vi "Get Target Method Path.vi"(7 "App Inst":refnum<vi>, 8 "error in (no error)":errorcluster, 10 "Target Method":string, 11 "Target Actor Path":path) -> (0 "error out":errorcluster, 2 "Target Method Path":path)   [LabVIEW 2020, in "Message Rescripter.lvlib"]
uses:
  Message Rescripter.lvlib
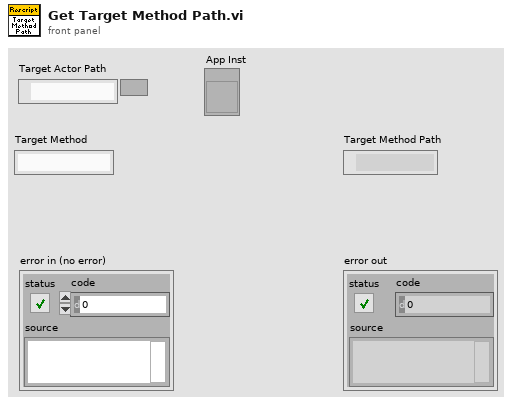
[diagram p1: front panel]
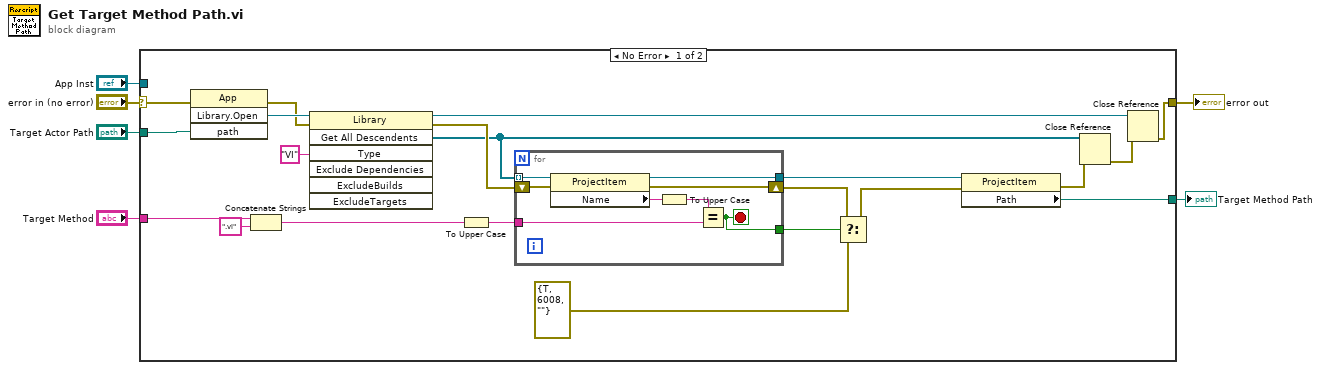
[diagram p0: block diagram]
diagram:
  n1 = case shown="No Error" "error in (no error)" {
    selector: "error in (no error)" -> [w14 w36]
    tunnel: "Target Actor Path" -> [w27 _]
    tunnel: "Target Method" -> [w24 _]
    tunnel: [w18 _] -> w4
    tunnel: [w15 w36] -> w2
    tunnel: "App Inst" -> [_ _]
    frame No Error {
      n2 = invoke class="App" method="Library.Open"(error in=w14, "path"=w27) -> (error out=w13:errorcluster, "Open Library"=w26:refnum<vi>)  [unwired: 2 in, 2 out]
      n3 = Concatenate Strings(w24, ".vi" ("string")) -> (w8:string)
      n4 = invoke class="Library" method="Get All Descendents"(reference=w26, error in=w13, "Type"="VI") -> (reference out=w17:refnum<vi>, error out=w21:errorcluster, "All Descendents"=w19:refnum<vi>[])  [unwired: 4 in, 4 out]
      n5 = To Upper Case(1:w8) -> (0:w23:string)
      n6 = for {
        tunnel: w19 -> [w34] mode=indexing
        tunnel: [w33] -> w22
        tunnel: w23 -> [w32]
        shift-right: [w30] -> w11
        shift-left: w21 -> [w31]
        tunnel: [w29] -> w12
        stop <- w29 stop-if-true
        n7 = property class="ProjectItem"(reference=w34, error in=w31) -> (reference out=w33:refnum<vi>, error out=w30:errorcluster, "Name"=w35:string)
        n8 = To Upper Case(1:w35) -> (0:w28:string)
        n9 = Equal?(x=w28, y=w32) -> (x = y?=w29:bool)
      }
      n10 = Select(t=w11, s=w12, f=errorcluster {"status"=TRUE, "code"=6008, "source"=""}) -> (s? t:f=w10:errorcluster)
      n11 = property class="ProjectItem"(reference=w22, error in=w10) -> (error out=w20:errorcluster, "Path"=w18:path)  [unwired: 1 out]
      n12 = Close Reference(reference=w19, error in (no error)=w20) -> (error out=w16:errorcluster)
      n13 = Close Reference(reference=w17, error in (no error)=w16) -> (error out=w15:errorcluster)
    }
    frame Error {
    }
  }
  "error out" <- w2
  "Target Method Path" <- w4
